vi "SetAttr Bool.vi"(8 "error in (no error)":errorcluster, 9 "Bool Value":bool, 10 "AttributeName":string, 11 "IMAQdx Actor in":refnum<class "IMAQdx Actor.lvclass">) -> (0 "error out":errorcluster, 3 "IMAQdx Actor out":refnum<class "IMAQdx Actor.lvclass">)   [LabVIEW 2020, in "IMAQdx Actor.lvlib" / "IMAQdx Actor.lvclass"]
uses:
  IMAQdx Actor.lvclass
  IMAQdx Actor.lvclass/IMAQdx Actor.ctl
  <resource>/objmgr/imaqdx.rc
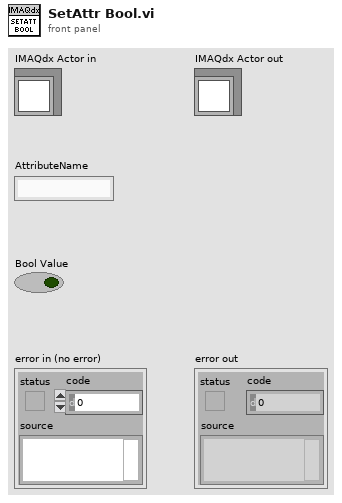
[diagram p1: front panel]
types:
  T1 = typedef "IMAQdx.ctl" = refnum<k21>
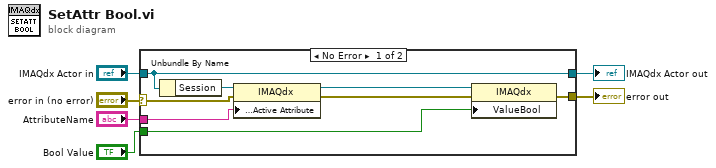
[diagram p0: block diagram]
diagram:
  n1 = case shown="No Error" "error in (no error)" {
    selector: "error in (no error)" -> [w8 w16]
    tunnel: [w7 w16] -> w5
    tunnel: [w14 w15] -> w3
    tunnel: "IMAQdx Actor in" -> [w14 w15]
    tunnel: "AttributeName" -> [w12 _]
    tunnel: "Bool Value" -> [w9 _]
    frame No Error {
      n2 = Unbundle By Name(w14) -> ("Session"=w13:T1)
      n3 = property class="IMAQdx"(reference=w13, error in=w8, "Camera Attributes:Active Attribute"=w12) -> (reference out=w10:T1, error out=w11:errorcluster)
      n4 = property class="IMAQdx"(reference=w10, error in=w11, "ValueBool"=w9) -> (error out=w7:errorcluster)  [unwired: 1 out]
    }
    frame Error {
    }
  }
  "error out" <- w5
  "IMAQdx Actor out" <- w3
